vi "CVT2ReferenceReadTest.vi"() -> (3 "Unit Test Framework Results":T1)   [LabVIEW 2013, in "UnitTests.lvlib"]
uses:
  UnitTests.lvlib
  <vilib>/utf/common/utf_test_result_troll.ctl
  <vilib>/utf/common/utf_test_result.ctl
  <vilib>/utf/common/utf_test_result_failure.ctl
  <vilib>/utf/common/utf_test_comparison_operators.ctl
  <vilib>/utf/common/utf_vi_tag.ctl
  <vilib>/NI/Current Value Table/Type Defs/Data Types.ctl
  <vilib>/NI/Current Value Table/DataTypes/I32_Read Index Set.vi
  <vilib>/NI/Current Value Table/FGVs/Tag Memory.vi
  <vilib>/NI/Current Value Table/Memory Block.vi
  <vilib>/NI/Current Value Table/DataTypes/I32_Memory Block.vi
  <vilib>/utf/NI_UnitTestFramework.lvlib
  <vilib>/NI/Current Value Table/Current Value Table.lvlib
panel:
  out "Values":i32[](array[numeric])
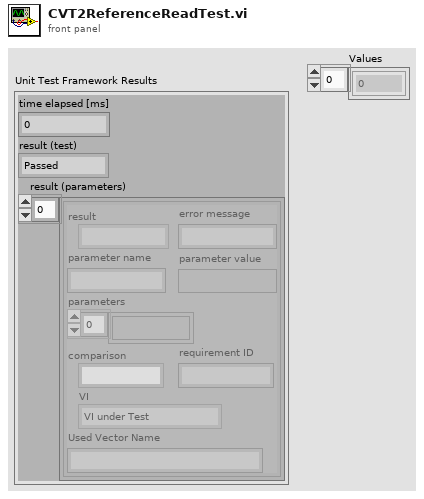
[diagram p1: front panel]
types:
  T1 = typedef "NI_UnitTestFramework.lvlib/utf_test_result_troll.ctl" = cluster{"time elapsed [ms]":u32, "result (test)":T2, "result (parameters)":T3[]}
  T2 = typedef "NI_UnitTestFramework.lvlib/utf_test_result.ctl" = enum16{"Passed", "Failed", "Error", "Skipped", "Not Processed"}
  T3 = typedef "NI_UnitTestFramework.lvlib/utf_test_result_failure.ctl" = cluster{"result":T2, "error message":string, "parameter name":string, "parameter value":variant, "parameters":variant[], "comparison":T4, "requirement ID":string, "VI":T5, "Used Vector Name":string}
  T4 = typedef "NI_UnitTestFramework.lvlib/utf_test_comparison_operators.ctl" = enum16{"=", "!=", ">", ">=", "<", "<=", "range", "symmetric tolerance", "asymmetric tolerance", "string contains", "string not contain", "array size", "string length", "array range", "by element", "array range (limit array)", "user-defined", "array contains", "array not contain", "vector length", "= (elm)", "!= (elm)", "= (case insensitive)", "!= (case insensitive)"}
  T5 = typedef "NI_UnitTestFramework.lvlib/utf_vi_tag.ctl" = enum16{"Setup VI", "VI under Test", "Teardown VI"}
  T6 = typedef "Current Value Table.lvlib/Data Types.ctl" = enum16{"Double", "Single", "I64", "I32", "I16", "I8", "U64", "U32", "U16", "U8", "String", "Boolean", "Array of U8", "Array of U16", "Array of U32", "Array of U64", "Array of I64", "Array of I32", "Array of I16", "Array of I8", "Array of Double", "Array of Single", "Array of Boolean", "Array of String"}
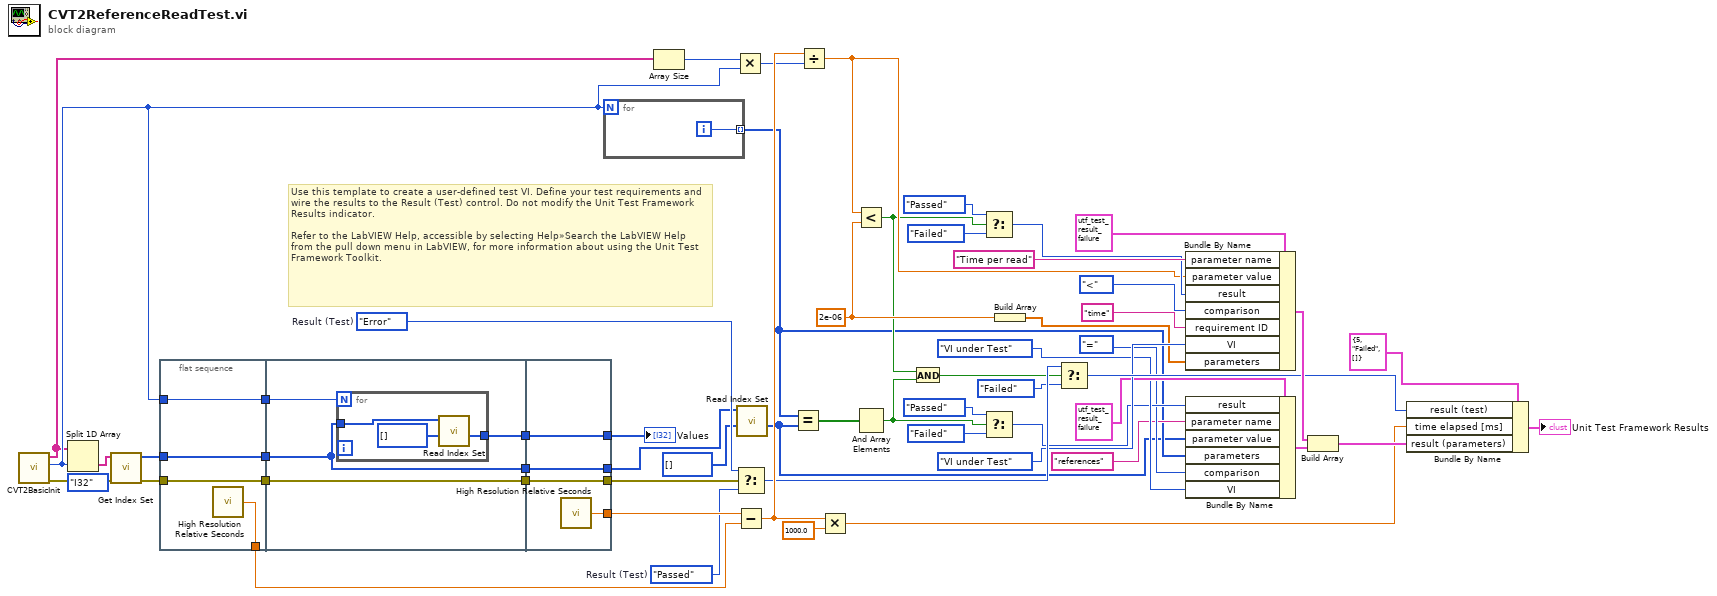
[diagram p0: block diagram]
diagram:
  w33 = 2e-06 ("y")
  w53 = utf_test_result."Error"  # Result (Test)
  w52 = utf_test_result."Passed"  # Result (Test)
  # "Use this template to create a user-defined test VI. Define your test requirements and wire the results to the Result (Test) control. Do not modify the Unit Test Framework Results indicator. \n\nRefer to the LabVIEW Help, accessible by selecting Help»Search the LabVIEW Help from the pull down menu in LabVIEW, for more information about using the Unit Test Framework Toolkit."
  n1 = call "CVT2BasicInit.vi"() -> ("error out"=w12:errorcluster, "Tags per type out"=w14:i32, "names"=w13:string[])  [unwired: 9 in]
  n2 = Split 1D Array(array=w13, index=w14) -> (second subarray=w2:string[])  [unwired: 1 out]
  n3 = call <vilib>:"Get Index Set.vi"("error in (no error)"=w12, "Expected Type"=Data_Types."I32", "Tag Names"=w2) -> ("error out"=w3:errorcluster, "Tag References"=w9:i32[])  [unwired: 7 in]
  n4 = flat-sequence {
    tunnel: [w62] -> w55
    tunnel: w3 -> [w60]
    tunnel: [w61] -> w47
    tunnel: w14 -> [w61]
    tunnel: [w60] -> w46
    tunnel: [w59] -> w10
    tunnel: w9 -> [w59]
    tunnel: w47 -> [w66]
    tunnel: w46 -> [w64]
    tunnel: [w65] -> w28
    tunnel: [w64] -> w11
    tunnel: w10 -> [w63]
    tunnel: [w63] -> w8
    tunnel: [w73] -> w56
    tunnel: [w72] -> w6
    tunnel: [w71] -> w27
    tunnel: w28 -> [w71]
    tunnel: w11 -> [w72]
    tunnel: [w70] -> w7
    tunnel: w8 -> [w70]
    frame #0 {
      n5 = call <vilib>:"High Resolution Relative Seconds.vi"() -> ("relative seconds"=w62:dbl)
    }
    frame #1 {
      n6 = for {
        N: w66 -> [_]
        tunnel: [w68] -> w65
        tunnel: w63 -> [w67]
        n7 = call-poly <vilib>:"Read Index Set.vi"("Default"=i32[] [], "Indices"=w67) -> ("Values"=w68:i32[])  [unwired: 9 in]
      }
    }
    frame #2 {
      n8 = call <vilib>:"High Resolution Relative Seconds.vi"() -> ("relative seconds"=w73:dbl)
    }
  }
  n9 = for {
    N: w14 -> [_]
    tunnel: [w74] -> w15 mode=indexing
    i -> [w74]
  }
  n10 = Array Size(array=w13) -> (size(s)=w26:i32)
  n11 = Multiply(x=w26, y=w14) -> (x*y=w25:i32)
  n12 = Select(t=w53, s=w6, f=w52) -> (s? t:f=w43:T2)
  n13 = Subtract(x=w56, y=w55) -> (x-y=w45:dbl)
  n14 = call-poly <vilib>:"Read Index Set.vi"("Default"=i32[] [], "Indices"=w7) -> ("Values"=w4:i32[])  [unwired: 9 in]
  n15 = Equal?(x=w15, y=w4) -> (x = y?=w17:bool[])
  n16 = Divide(x=w45, y=w25) -> (x/y=w36:dbl)
  n17 = Multiply(x=w45, y=1000.0) -> (x*y=w48:dbl)
  n18 = Less?(x=w36, y=w33) -> (x < y?=w29:bool)
  n19 = And Array Elements(Boolean array=w17) -> (logical AND=w16:bool)
  n20 = And(x=w29, y=w16) -> (x .and. y?=w30:bool)
  n21 = Select(t=utf_test_result."Passed" ("result"), s=w29, f=utf_test_result."Failed" ("result")) -> (s? t:f=w37:T2)
  n22 = Select(t=utf_test_result."Passed" ("result"), s=w16, f=utf_test_result."Failed" ("result")) -> (s? t:f=w20:T2)
  n23 = Build Array(w33) -> (w32:dbl[])
  n24 = Select(t=w43, s=w30, f=utf_test_result."Failed") -> (s? t:f=w41:T2)
  n25 = Bundle By Name(cluster=T3 {"result"=enum."Passed", "error message"="", "parameter name"="", "parameter value"=variant, "parameters"=[], "comparison"=enum."=", "requirement ID"="", "VI"=enum."Setup VI", "Used Vector Name"=""} ("Unit Test Framework - result (parameters)"), "parameter name"="Time per read", "parameter value"=w36, "result"=w37, "comparison"=utf_test_comparison_operators."<", "requirement ID"="time", "VI"=utf_vi_tag."VI under Test", "parameters"=w32) -> (w51:T3)
  n26 = Bundle By Name(cluster=T3 {"result"=enum."Passed", "error message"="", "parameter name"="", "parameter value"=variant, "parameters"=[], "comparison"=enum."=", "requirement ID"="", "VI"=enum."Setup VI", "Used Vector Name"=""} ("Unit Test Framework - result (parameters)"), "result"=w20, "parameter name"="references" ("format string"), "parameter value"=w4, "parameters"=w15, "comparison"=utf_test_comparison_operators."=", "VI"=utf_vi_tag."VI under Test") -> (w31:T3)
  n27 = Build Array(w51, w31) -> (w50:T3[])
  n28 = Bundle By Name(cluster=T1 {"time elapsed [ms]"=5, "result (test)"=enum."Failed", "result (parameters)"=[]} ("Unit Test Framework - Result"), "result (test)"=w41, "time elapsed [ms]"=w48, "result (parameters)"=w50) -> (→"Unit Test Framework Results":T1)
  "Values" <- w27
